vi "Send Update_RawActPosition.vi"(7 "Message Priority (Normal)":T1=enum."Normal", 8 "error in (no error)":errorcluster, 10 "RawActPosition?":dbl, 11 "Message Enqueuer":refnum<class "Message Enqueuer.lvclass">) -> (0 "error out":errorcluster, 3 "Message Enqueuer out":refnum<class "Message Enqueuer.lvclass">)   [LabVIEW 2015, in "CS++Motor.lvlib" / "Update_RawActPosition Msg.lvclass"]
doc: "Sends the <B>CS++Motor.lvlib:Update_RawActPosition Msg.lvclass</B> message.\n\n<B>CS++Motor.lvlib:CS++Motor.lvclass:Update_RawActPosition.vi</B> Description:\n\nThis VI is executed via the corresponding Monitor Actor and delivers the information abot the Raw Act Position of an axis."
uses:
  Update_RawActPosition Msg.lvclass
  <vilib>/ActorFramework/Message Enqueuer/Message Enqueuer.lvclass
  <vilib>/ActorFramework/Message Enqueuer/Message Priority.ctl
  Update_RawActPosition Msg.lvclass/Update_RawActPosition Msg.ctl
  <vilib>/ActorFramework/Message Enqueuer/Message Enqueuer.lvclass/Message Enqueuer.ctl
  <vilib>/ActorFramework/Message Priority Queue/Priority Enqueue.vi
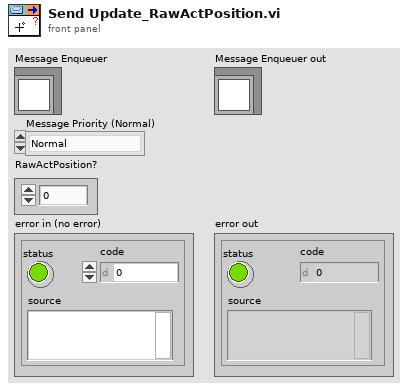
[diagram p1: front panel]
types:
  T1 = typedef "Actor Framework.lvlib/Message Enqueuer.lvclass/Message Priority.ctl" = enum16{"Low", "Normal", "High"}
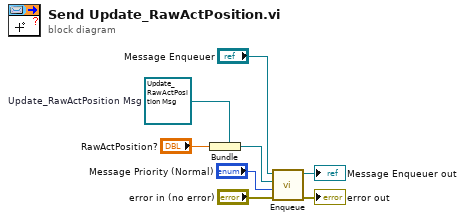
[diagram p0: block diagram]
diagram:
  w2 = refnum<class "Update_RawActPosition Msg.lvclass"> refnum  # Update_RawActPosition Msg
  n1 = Bundle(cluster=w2, "RawActPosition?") -> (w5:refnum<class "Update_RawActPosition Msg.lvclass">)
  n2 = call <vilib>:"Enqueue.vi"("error in (no error)"="error in (no error)", "Message Priority (Normal)"="Message Priority (Normal)", "Message"=w5, "Message Enqueuer in"="Message Enqueuer") -> ("error out"=→"error out":errorcluster, "Message Enqueuer out"=→"Message Enqueuer out":refnum<class "Message Enqueuer.lvclass">)  [unwired: 6 in]
